vi "SaveNewServerRef.vi"(2 "error":errorcluster, 3 "vi reference":refnum<vi>, 4 "Baxter in":T2) -> (0 "Active Topics":T1(array[cluster]), 1 "Baxter out":T2)   [LabVIEW 2013]
uses:
  _ROSControl.ctl
  _ROSDirection.ctl
  _ROSDefinition.vi
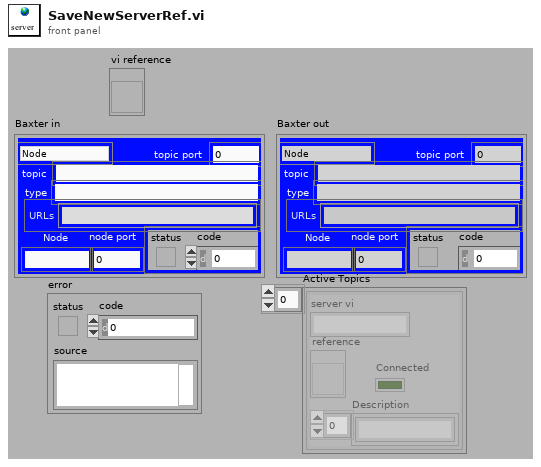
[diagram p1: front panel]
types:
  T1 = cluster{"server vi":string, "reference":refnum<vi>, "Description":string[], "Connected":bool}[]
  T2 = typedef "_ROSControl.ctl" = cluster{"topic port":u16, "Node":string, "topic":string, "type":string, "node port":u32, "error ":errorcluster, "Direction":T3, "APIs":string[]}
  T3 = typedef "_ROSDirection.ctl" = enum16{"Node", "Publisher", "Subscriber", "Service Client"}
  T4 = cluster{"vi name":string, "vi reference":refnum<vi>, string[], bool}
  T5 = cluster{"vi name":string, "vi reference":refnum<vi>, "Description":string[], "Connected":bool}[]
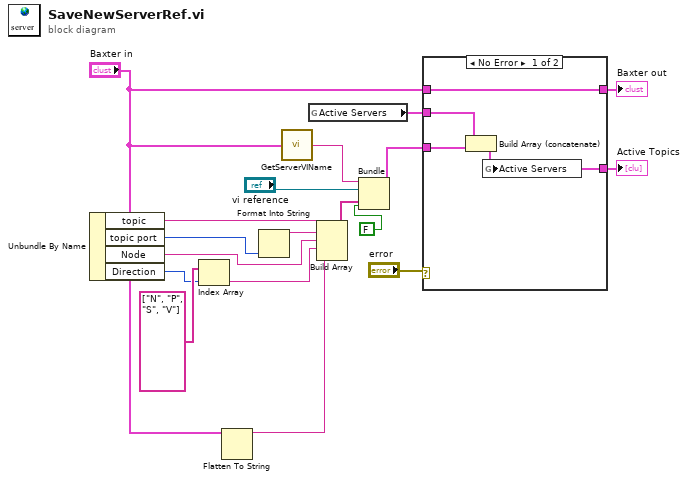
[diagram p0: block diagram]
diagram:
  n1 = Unbundle By Name("Baxter in") -> ("topic"=w7:string, "topic port"=w13:u16, "Node"=w8:string, "Direction"=w10:T3)
  n2 = Index Array(array=string[] ["N", "P", "S", "V"], index=w10) -> (element=w9:string)
  n3 = Flatten To String(anything="Baxter in") -> (data string=w2:string)  [unwired: 3 in, 2 out]
  n4 = Format Into String(w13) -> (resulting string=w12:string)  [unwired: 3 in, 1 out]
  n5 = call "GetServerVIName.vi"("Baxter"="Baxter in") -> ("vi name"=w16:string)
  n6 = global read "_ROSDefinition.vi" "Active Servers"() -> (w4:T1)
  n7 = Build Array(w7, w12, w8, w9, w2) -> (w6:string[])
  n8 = Bundle("vi name"=w16, "vi reference"="vi reference", w6, FALSE) -> (w14:T4)  [unwired: 1 in]
  n9 = case shown="No Error" "error" {
    tunnel: [w21 w24] -> w17
    tunnel: "Baxter in" -> [w21 w24]
    tunnel: w14 -> [w22 _]
    tunnel: [w20 w23] -> w5
    tunnel: w4 -> [w19 w23]
    frame No Error {
      n10 = Build Array (concatenate)(w19, w22) -> (w20:T5)
      n11 = global write "_ROSDefinition.vi" "Active Servers"(w20) -> ()
    }
    frame Error {
    }
  }
  "Baxter out" <- w17
  "Active Topics" <- w5
